vi "Add NI-XNET CAN Hardware_Add Outgoing Event Triggered.vi"(6 "Sporadic Frames":T2[](array[typedef]) {"Phase" items=["Unchanged", "Reset"]; "TriggerType" items=["ChannelValueChange", "TriggerChannelNotZero", "ChannelValueChangeOrTriggerChannelNotZero"]}, 7 "SysDef Ref":T1, 8 "error in (no error)":errorcluster, 9 "ClusterName":string, 10 "Owning Database":refnum<k24>, 11 "CAN Port":refnum<k24>) -> (0 "error out":errorcluster, 3 "CAN Port out":refnum<k24>)   [LabVIEW 2019, in "Simple SysDef API.lvlib"]
uses:
  <userlib>/SimpleSysDef/Simple SysDef API.lvlib
  <userlib>/SimpleSysDef/_SubVIs/Add NI-XNET CAN Hardware_Sporadic Frame Settings.ctl
  <userlib>/SimpleSysDef/_SubVIs/Add NI-XNET CAN Hardware_Frame Settings.ctl
  <userlib>/SimpleSysDef/_SubVIs/Add NI-XNET CAN Hardware_Signal Settings.ctl
  NationalInstruments.VeriStand.SystemDefinitionAPI
  <userlib>/SimpleSysDef/_SubVIs/System Definition Reference.ctl
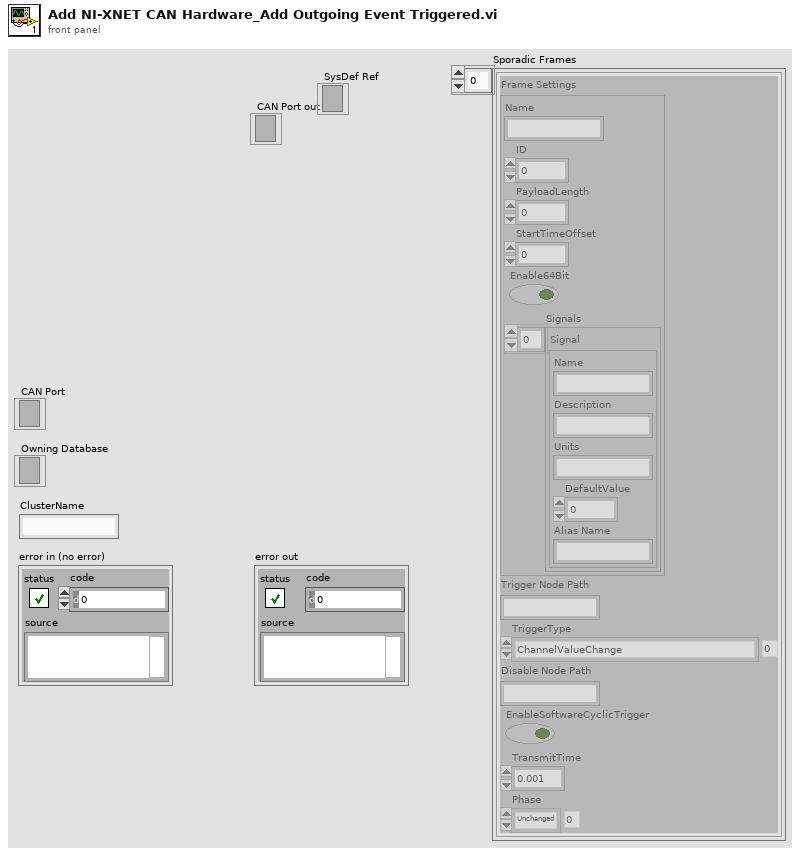
[diagram p1: front panel]
types:
  T1 = typedef "Simple SysDef API.lvlib/System Definition Reference.ctl" = refnum<k24>
  T2 = typedef "Simple SysDef API.lvlib/Add NI-XNET CAN Hardware_Sporadic Frame Settings.ctl" = cluster{"Frame Settings":T3, "Trigger Node Path":string, "TriggerType":i32, "Disable Node Path":string, "EnableSoftwareCyclicTrigger":bool, "TransmitTime":dbl, "Phase":i32}
  T3 = typedef "Simple SysDef API.lvlib/Add NI-XNET CAN Hardware_Frame Settings.ctl" = cluster{"Name":string, "ID":u32, "PayloadLength":u32, "StartTimeOffset":dbl, "Enable64Bit":bool, "Signals":T4[]}
  T4 = typedef "Simple SysDef API.lvlib/Add NI-XNET CAN Hardware_Signal Settings.ctl" = cluster{"Name":string, "Description":string, "Units":string, "DefaultValue":dbl, "Alias Name":string}
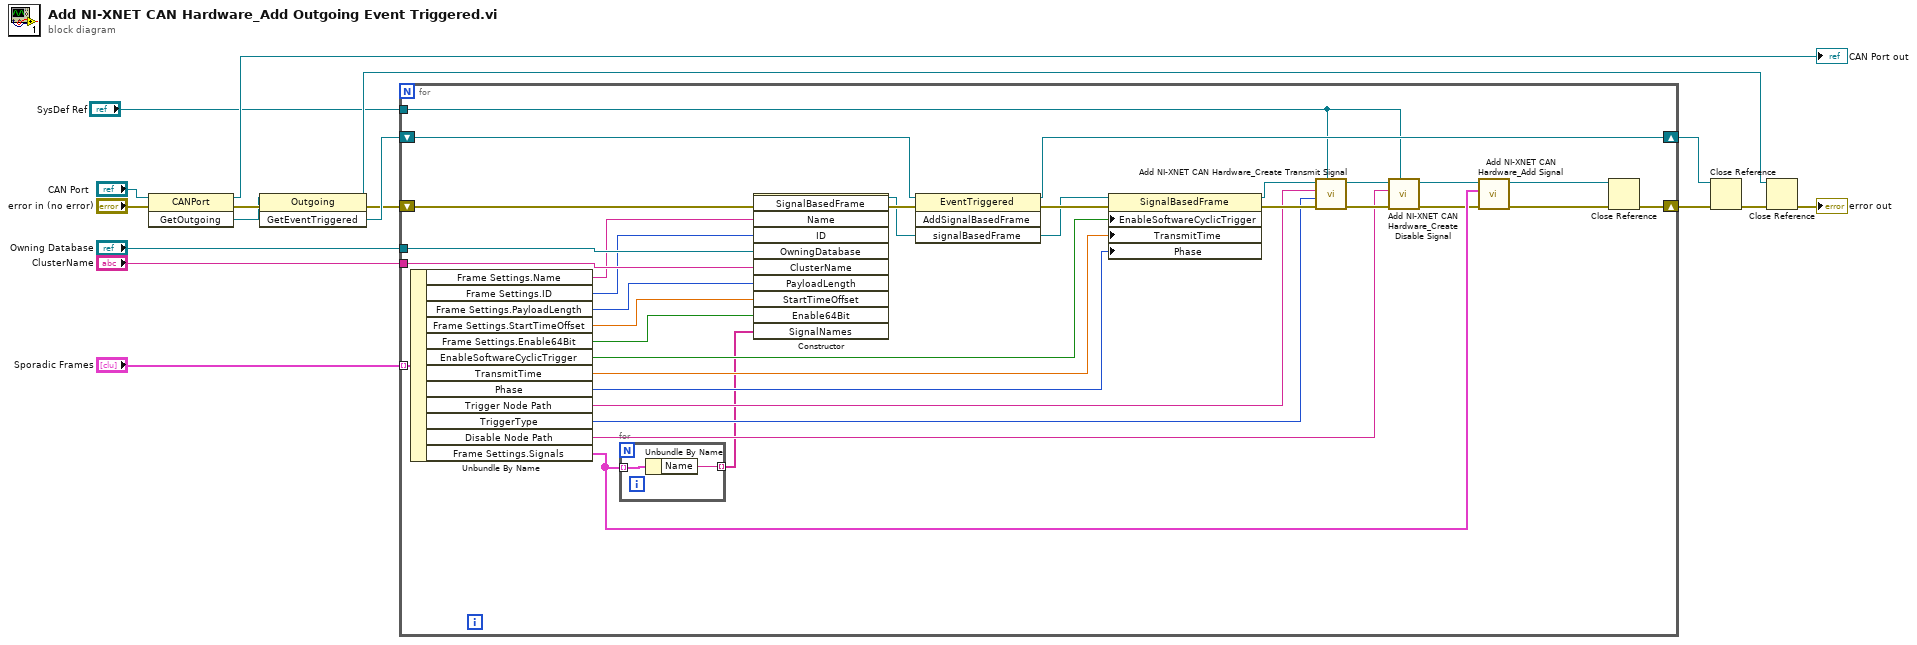
[diagram p0: block diagram]
diagram:
  n1 = invoke class="CANPort" method="GetOutgoing"(reference="CAN Port", error in="error in (no error)") -> (reference out=→"CAN Port out":refnum<k24>, error out=w8:errorcluster, "GetOutgoing"=w1:refnum<k24>)  [unwired: 1 in]
  n2 = invoke class="Outgoing" method="GetEventTriggered"(reference=w1, error in=w8) -> (reference out=w5:refnum<k24>, error out=w12:errorcluster, "GetEventTriggered"=w13:refnum<k24>)  [unwired: 1 in]
  n3 = for {
    shift-right: [w35] -> w10
    shift-left: w12 -> [w47]
    shift-right: [w27] -> w11
    shift-left: w13 -> [w46]
    tunnel: "Sporadic Frames" -> [w43] mode=indexing
    tunnel: "Owning Database" -> [w45]
    tunnel: "ClusterName" -> [w44]
    tunnel: "SysDef Ref" -> [w24]
    n4 = Unbundle By Name(w43) -> ("Frame Settings.Name"=w42:string, "Frame Settings.ID"=w41:u32, "Frame Settings.PayloadLength"=w40:u32, "Frame Settings.StartTimeOffset"=w39:dbl, "Frame Settings.Enable64Bit"=w38:bool, "EnableSoftwareCyclicTrigger"=w30:bool, "TransmitTime"=w29:dbl, "Phase"=w28:i32, "Trigger Node Path"=w26:string, "TriggerType"=w25:i32, "Disable Node Path"=w23:string, "Frame Settings.Signals"=w21:T4[])
    n5 = for {
      tunnel: w21 -> [w50] mode=indexing
      tunnel: [w49] -> w22 mode=indexing
      n6 = Unbundle By Name(w50) -> ("Name"=w49:string)
    }
    n7 = constructor class="SignalBasedFrame"(error in=w47, "Name"=w42, "ID"=w41, "OwningDatabase"=w45, "ClusterName"=w44, "PayloadLength"=w40, "StartTimeOffset"=w39, "Enable64Bit"=w38, "SignalNames"=w22) -> (reference out=w32:refnum<k24>, error out=w48:errorcluster)  [unwired: 2 in, 9 out]
    n8 = invoke class="EventTriggered" method="AddSignalBasedFrame"(reference=w46, error in=w48, "signalBasedFrame"=w32) -> (reference out=w27:refnum<k24>, error out=w34:errorcluster)  [unwired: 1 in, 2 out]
    n9 = property class="SignalBasedFrame"(reference=w32, error in=w34, "EnableSoftwareCyclicTrigger"=w30, "TransmitTime"=w29, "Phase"=w28) -> (reference out=w31:refnum<k24>, error out=w33:errorcluster)
    n10 = call <userlib>:"Add NI-XNET CAN Hardware_Create Transmit Signal.vi"("SysDef Ref"=w24, "error in (no error)"=w33, "TriggerType"=w25, "Trigger Node Path"=w26, "Frame Based Signal"=w31) -> ("error out"=w36:errorcluster, "Frame Based Signal out"=w37:refnum<k24>)  [unwired: 5 in]
    n11 = call <userlib>:"Add NI-XNET CAN Hardware_Create Disable Signal.vi"("SysDef Ref"=w24, "error in (no error)"=w36, "Disable Node Path"=w23, "Signal Based Frame"=w37) -> ("error out"=w20:errorcluster, "Signal Based Frame out"=w18:refnum<k24>)  [unwired: 6 in]
    n12 = call <userlib>:"Add NI-XNET CAN Hardware_Add Signal.vi"("error in (no error)"=w20, "Signals"=w21, "Frame Ref"=w18) -> ("error out"=w19:errorcluster, "Frame Ref out"=w17:refnum<k24>)  [unwired: 7 in]
    n13 = Close Reference(reference=w17, error in (no error)=w19) -> (error out=w35:errorcluster)
  }
  n14 = Close Reference(reference=w11, error in (no error)=w10) -> (error out=w7:errorcluster)
  n15 = Close Reference(reference=w5, error in (no error)=w7) -> (error out=→"error out":errorcluster)
